vi "Config_Populate.vi"(8 "error in (no error)":errorcluster, 11 "Config Ref In":T1) -> (0 "error out":errorcluster, 3 "refnum out":T1)   [LabVIEW 2021]
uses:
  <vilib>/Utility/config.llb/Config Data RefNum.ctl
  Config_Cluster.ctl
  Mode_Enum.ctl
  <vilib>/Utility/config.llb/Write Key (Path).vi
  <vilib>/Utility/config.llb/Write Key (String).vi
  <vilib>/Utility/config.llb/NI_LVConfig.lvlib
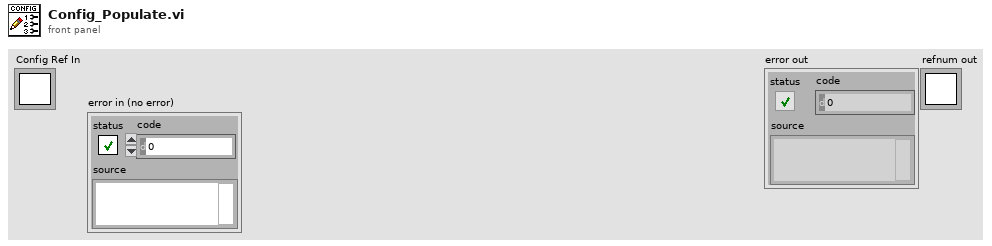
[diagram p1: front panel]
types:
  T1 = typedef "NI_LVConfig.lvlib/Config Data RefNum.ctl" = refnum<k1>
  T2 = typedef "Config_Cluster.ctl" = cluster{"General":cluster{"Config.ini":path, "Default Logging Path":path}, "Hardware":cluster{"Measure Rate (1/s)":i32, "HP DMM VISA":refnum<visa-resource-name>, "LS 335 VISA":refnum<visa-resource-name>, "HP DM":cluster{"Range":enum16{"Autorange", "30mV", "300mV", "3V", "30V"}, "Autozero":bool, "Display":enum16{"3 1/2 Digit", "4 1/2 Digit", "5 1/2 Digit"}, "Blank LCD":bool}}, "Operation":cluster{"Operation Mode":T3, "Status":string, "NewLog?":bool, "OvenWarn":bool}}
  T3 = typedef "Mode_Enum.ctl" = enum16{"OvenNRDY", "Logging", "Idle-Off", "Idle"}
  T4 = cluster{"Config.ini":path, "Default Logging Path":path}
  T5 = cluster{"Measure Rate (1/s)":i32, "HP DMM VISA":refnum<visa-resource-name>, "LS 335 VISA":refnum<visa-resource-name>, "HP DM":cluster{"Range":enum16{"Autorange", "30mV", "300mV", "3V", "30V"}, "Autozero":bool, "Display":enum16{"3 1/2 Digit", "4 1/2 Digit", "5 1/2 Digit"}, "Blank LCD":bool}}
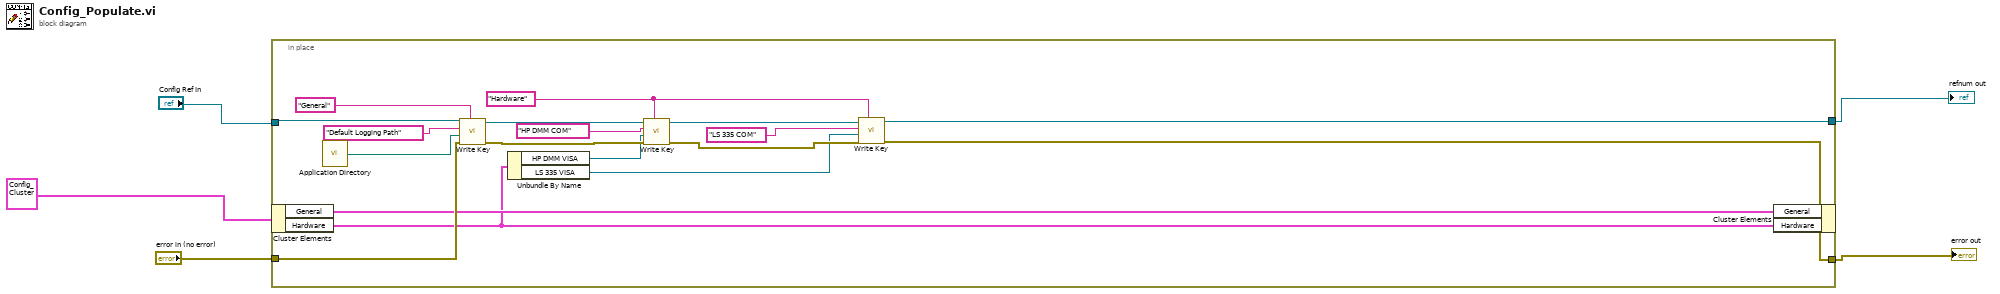
[diagram p0: block diagram]
diagram:
  n1 = in-place {
    in-place-border: "Config Ref In" -> [w23]
    in-place-border: "error in (no error)" -> [w22]
    in-place-border: [w7] -> w2
    in-place-border: [w10] -> w1
    w9 = "Hardware" ("section")
    n2 = in-place-cluster #1(T2 {"General"={"Config.ini"=path "", "Default Logging Path"=path ""}, "Hardware"={"Measure Rate (1/s)"=0, "HP DMM VISA"="", "LS 335 VISA"="", "HP DM"={"Range"=enum."Autorange", "Autozero"=FALSE, "Display"=enum."3 1/2 Digit", "Blank LCD"=FALSE}}, "Operation"={"Operation Mode"=enum."Logging", "Status"="", "NewLog?"=FALSE, "OvenWarn"=FALSE}} ("Configuration Cluster")) -> ("General"=w19:T4, "Hardware"=w18:T5)
    n3 = call <vilib>:"Application Directory.vi"() -> ("Application Directory"=w11:path)
    n4 = call-poly <vilib>:"Write Key.vi"("section"="General", "error in (no error)"=w22, "value"=w11, "key"="Default Logging Path", "refnum"=w23) -> ("error out"=w17:errorcluster, "refnum out"=w20:T1)  [unwired: 4 in, 1 out]
    n5 = Unbundle By Name(w18) -> ("HP DMM VISA"=w15:refnum<visa-resource-name>, "LS 335 VISA"=w6:refnum<visa-resource-name>)
    n6 = call-poly <vilib>:"Write Key.vi"("section"=w9, "error in (no error)"=w17, "value"=w15, "key"="HP DMM COM", "refnum"=w20) -> ("error out"=w12:errorcluster, "refnum out"=w13:T1)  [unwired: 4 in, 1 out]
    n7 = call-poly <vilib>:"Write Key.vi"("section"=w9, "error in (no error)"=w12, "value"=w6, "key"="LS 335 COM", "refnum"=w13) -> ("error out"=w7:errorcluster, "refnum out"=w10:T1)  [unwired: 4 in, 1 out]
    n8 = in-place-cluster #1("General"=w19, "Hardware"=w18) -> ()  [unwired: 1 out]
  }
  "error out" <- w2
  "refnum out" <- w1
